vi "ExtendedKalmanFilter_Reset.vi"(11 "in ExtendedKalmanFiilter":T1) -> (3 "out ExtendedKalmanFiilter":T1)   [LabVIEW 2019, in "Trajectory_Library.lvlib"]
doc: "Resets the filter.\n \nInputs:\n - inExtendedKalmanFIlter -- filter data cluster\n\nReturns:\n - outExtendedKalmanFIlter -- updated filter data cluster"
uses:
  Trajectory_Library.lvlib
  TypeDef/EXTENDED_KALMAN_FILTER.ctl
  <vilib>/Analysis/Matrix/Datatypes/RealMatrix.ctl
  <vilib>/Analysis/Matrix/NI_Matrix.lvlib
panel:
  # "State Estimate <Statess,1>"
  # "<States, States>"
  # "<States, States>"
  # "<Statess,  States>"
  # "<Outputs, Outputs>"
  # "State Estimate <Statess,1>"
  # "<States, States>"
  # "<States, States>"
  # "<Statess,  States>"
  # "<Outputs, Outputs>"
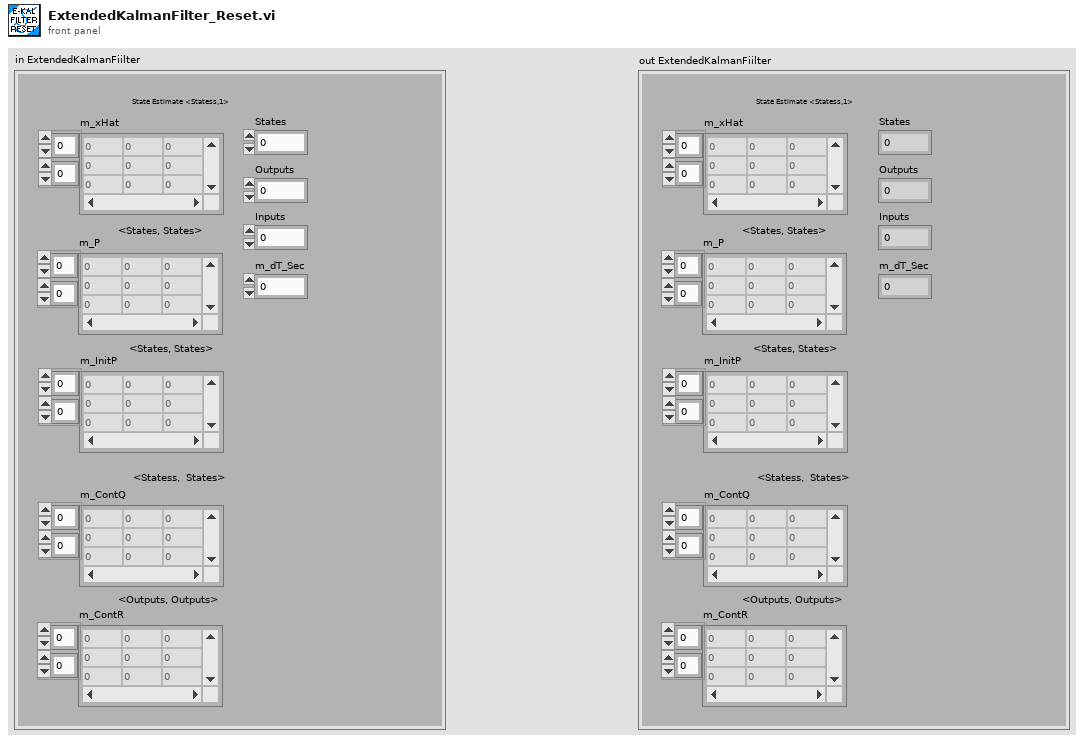
[diagram p1: front panel]
types:
  T1 = typedef "Trajectory_Library.lvlib/EXTENDED_KALMAN_FILTER.ctl" = cluster{"m_P":T2, "m_xHat":T2, "States":i32, "Outputs":i32, "m_ContR":T2, "m_ContQ":T2, "m_dT_Sec":dbl, "Inputs":i32, "m_InitP":T2}
  T2 = typedef "NI_Matrix.lvlib/RealMatrix.ctl" = dbl[][]
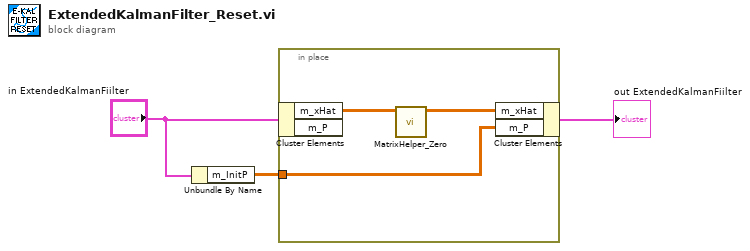
[diagram p0: block diagram]
diagram:
  n1 = Unbundle By Name("in ExtendedKalmanFiilter") -> ("m_InitP"=w1:T2)
  n2 = in-place {
    in-place-border: w1 -> [w4]
    n3 = in-place-cluster #1("in ExtendedKalmanFiilter") -> ("m_xHat"=w6:T2)  [unwired: 1 out]
    n4 = call "MatrixHelper_Zero.vi"("input matrix"=w6) -> ("output matrix"=w5:T2)  [unwired: 10 in]
    n5 = in-place-cluster #1("m_xHat"=w5, "m_P"=w4) -> (→"out ExtendedKalmanFiilter":T1)
  }
